vi "GEA2 Send and Receive Message.vi"(0 "GEA2 Reference In":refnum<k24>, 1 "Input Data":T1 {"Command" format="%02x"; "Destination" format="%02x"; "Source" format="%02x"}, 2 "Read Timeout":u32=500, 5 "Expected Command":string=".*", 7 "Expected Data":string=".*", 11 "Error In":errorcluster) -> (4 "GEA2 Reference Out":refnum<k24>, 6 "Raw Data Out":string, 8 "Converted Data Out":T2 {"CRC" format="%04x"; "Length" format="%02x"; "Command" format="%02x"; "Destination" format="%02x"; "Source" format="%02x"}, 15 "Error Out":errorcluster)   [LabVIEW 2014, in "GEA2_Toolkit.lvlib"]
doc: "This VI accepts an event registration input. The input event is generated every time a message is present on the GEA2 bus. When an event is detected the event structure exectures and the output of this VI contains source and destination address as well as the command and data."
uses:
  library/GEA2_Toolkit.lvlib
  C:/Automation/DLLs/PC Tools .NET/GeaCommunication.dll
  Automation/DLLs/PC Tools .NET/GeaCommunication.dll
  type defs/Data Out.ctl
  type defs/Data In.ctl
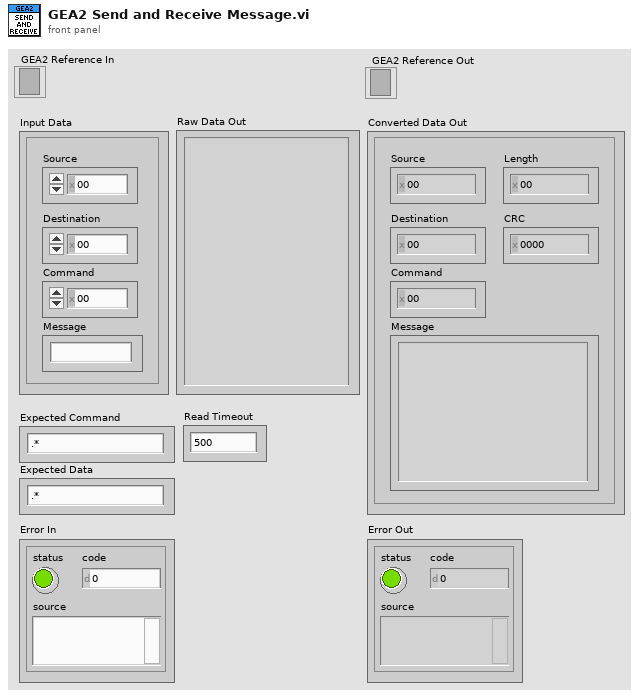
[diagram p1: front panel]
types:
  T1 = typedef "GEA2_Toolkit.lvlib/Data In.ctl" = cluster{"Source":u8, "Destination":u8, "Command":u8, "Message":string}
  T2 = typedef "GEA2_Toolkit.lvlib/Data Out.ctl" = cluster{"Source":u8, "Destination":u8, "Command":u8, "Length":u8, "CRC":u16, "Message":string}
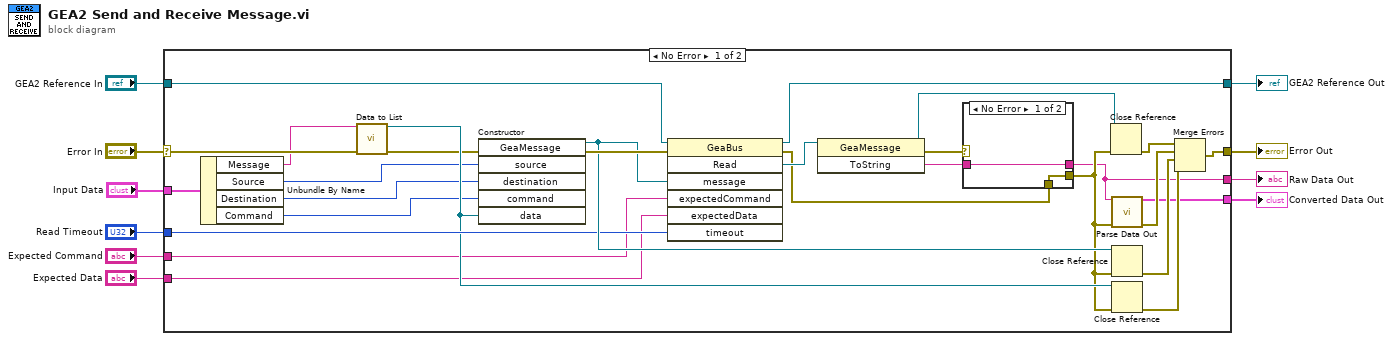
[diagram p0: block diagram]
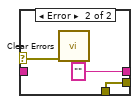
[diagram p2: hidden frame]
diagram:
  n1 = case shown="No Error" "Error In" {
    selector: "Error In" -> [w28 w44]
    tunnel: "GEA2 Reference In" -> [w27 w45]
    tunnel: [w11 _] -> w4
    tunnel: [w26 w45] -> w7
    tunnel: [w34 w44] -> w9
    tunnel: "Read Timeout" -> [w33 _]
    tunnel: [w12 _] -> w5
    tunnel: "Expected Data" -> [w21 _]
    tunnel: "Expected Command" -> [w20 _]
    tunnel: "Input Data" -> [w19 _]
    frame No Error {
      n2 = Unbundle By Name(w19) -> ("Message"=w18:string, "Source"=w17:u8, "Destination"=w16:u8, "Command"=w15:u8)
      n3 = call "Data to List.vi"("Data String In"=w18, "error in"=w28) -> ("Data List Out"=w30:refnum<k24>, "error out"=w29:errorcluster)  [unwired: 12 in]
      n4 = constructor class="GeaMessage"(error in=w29, "source"=w17, "destination"=w16, "command"=w15, "data"=w30) -> (reference out=w35:refnum<k24>, error out=w37:errorcluster)  [unwired: 2 in, 5 out]
      n5 = invoke class="GeaBus" method="Read"(reference=w27, error in=w37, "message"=w35, "expectedCommand"=w20, "expectedData"=w21, "timeout"=w33) -> (reference out=w26:refnum<k24>, error out=w14:errorcluster, "Read"=w38:refnum<k24>)  [unwired: 1 in, 4 out]
      n6 = invoke class="GeaMessage" method="ToString"(reference=w38) -> (reference out=w36:refnum<k24>, error out=w32:errorcluster, "ToString"=w31:string)  [unwired: 2 in]
      n7 = case shown="No Error" w32 {
        selector: w32 -> [_ w42]
        tunnel: w31 -> [w40 _]
        tunnel: [w40 "" ("ToString")] -> w12
        tunnel: [w39 w41] -> w13
        tunnel: w14 -> [w39 w41]
        frame No Error {
        }
        frame Error {
          n8 = call <vilib>:"Clear Errors.vi"("error in (no error)"=w42) -> ()  [unwired: 5 in, 2 out]
        }
      }
      n9 = Close Reference(reference=w36, error in (no error)=w13) -> (error out=w25:errorcluster)
      n10 = call "Parse Data Out.vi"("Raw Data In"=w12, "Error In"=w13) -> ("Data Out"=w11:T2, "Error Out"=w24:errorcluster)  [unwired: 12 in]
      n11 = Close Reference(reference=w35, error in (no error)=w13) -> (error out=w23:errorcluster)
      n12 = Close Reference(reference=w30, error in (no error)=w13) -> (error out=w22:errorcluster)
      n13 = Merge Errors(w25, w24, w23, w22) -> (w34:errorcluster)
    }
    frame Error {
    }
  }
  "Raw Data Out" <- w5
  "Error Out" <- w9
  "GEA2 Reference Out" <- w7
  "Converted Data Out" <- w4
